vi "getTiming.vi"(8 "error in (no error)":errorcluster, 11 "CameraSettingsManager.lvclass in":refnum<class "CameraSettingsManager.lvclass">) -> (0 "error out":errorcluster, 2 "Timing":T1={"shutter Open Time"=20.0, "Shutter Close Time"=20.0, "Exposure Time"=0.02, " AccumulatedCycleTime"=0.0, " KineticCycleTime"=0.0, "Number of Accumulations"=1.0, "Number in Kinetic Series "=1.0, "Shutter Mode"=0.0}, 3 "CameraSettingsManager.lvclass out":refnum<class "CameraSettingsManager.lvclass">)   [LabVIEW 2011, in "Tools.lvlib" / "Settings.lvlib" / "CameraSettingsManager.lvclass"]
uses:
  CameraSettingsManager.lvclass
  CameraSettingsManager.lvclass/CameraSettingsManager.ctl
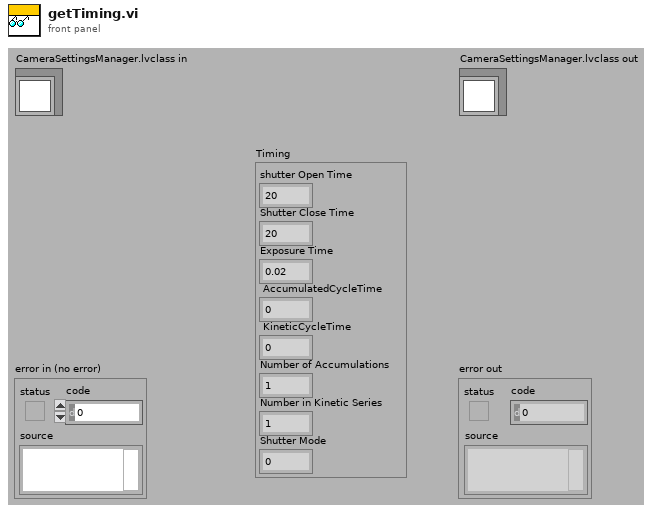
[diagram p1: front panel]
types:
  T1 = cluster{"shutter Open Time":dbl, "Shutter Close Time":dbl, "Exposure Time":dbl, " AccumulatedCycleTime":dbl, " KineticCycleTime":dbl, "Number of Accumulations":dbl, "Number in Kinetic Series ":dbl, "Shutter Mode":dbl}
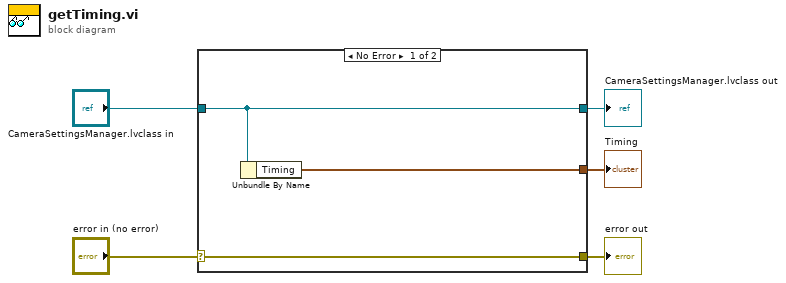
[diagram p0: block diagram]
diagram:
  n1 = case shown="No Error" "error in (no error)" {
    selector: "error in (no error)" -> [w8 w9]
    tunnel: [w8 w9] -> w4
    tunnel: [w7 w10] -> w2
    tunnel: "CameraSettingsManager.lvclass in" -> [w7 w10]
    tunnel: [w6 _] -> w1
    frame No Error {
      n2 = Unbundle By Name(w7) -> ("Timing"=w6:T1)
    }
    frame Error {
    }
  }
  "error out" <- w4
  "CameraSettingsManager.lvclass out" <- w2
  "Timing" <- w1
